vi "read_analog_inputs_from_telemetry.vi"(8 "error_in":errorcluster, 10 "channel_count":i32, 11 "paramUnicorn in":T1) -> (0 "error_out":errorcluster, 2 "values":sgl[](array[numeric]), 3 "paramUnicorn out":T1)   [LabVIEW 2017]
uses:
  Unicorn Labview Library/Control/unicorn_Param.ctl
  Unicorn Labview Library/Control/unicorn_conn.ctl
  Unicorn Labview Library/Control/unicorn_JSON.ctl
  Unicorn Labview Library/Control/unicorn_ParamInt.ctl
  Unicorn Labview Library/Control/unicorn_Telemetry.ctl
  Unicorn Labview Library/Control/unicorn_Table.ctl
  Unicorn Labview Library/Control/unicorn_ParamFloat.ctl
  Unicorn Labview Library/Unicorn Library.lvlib
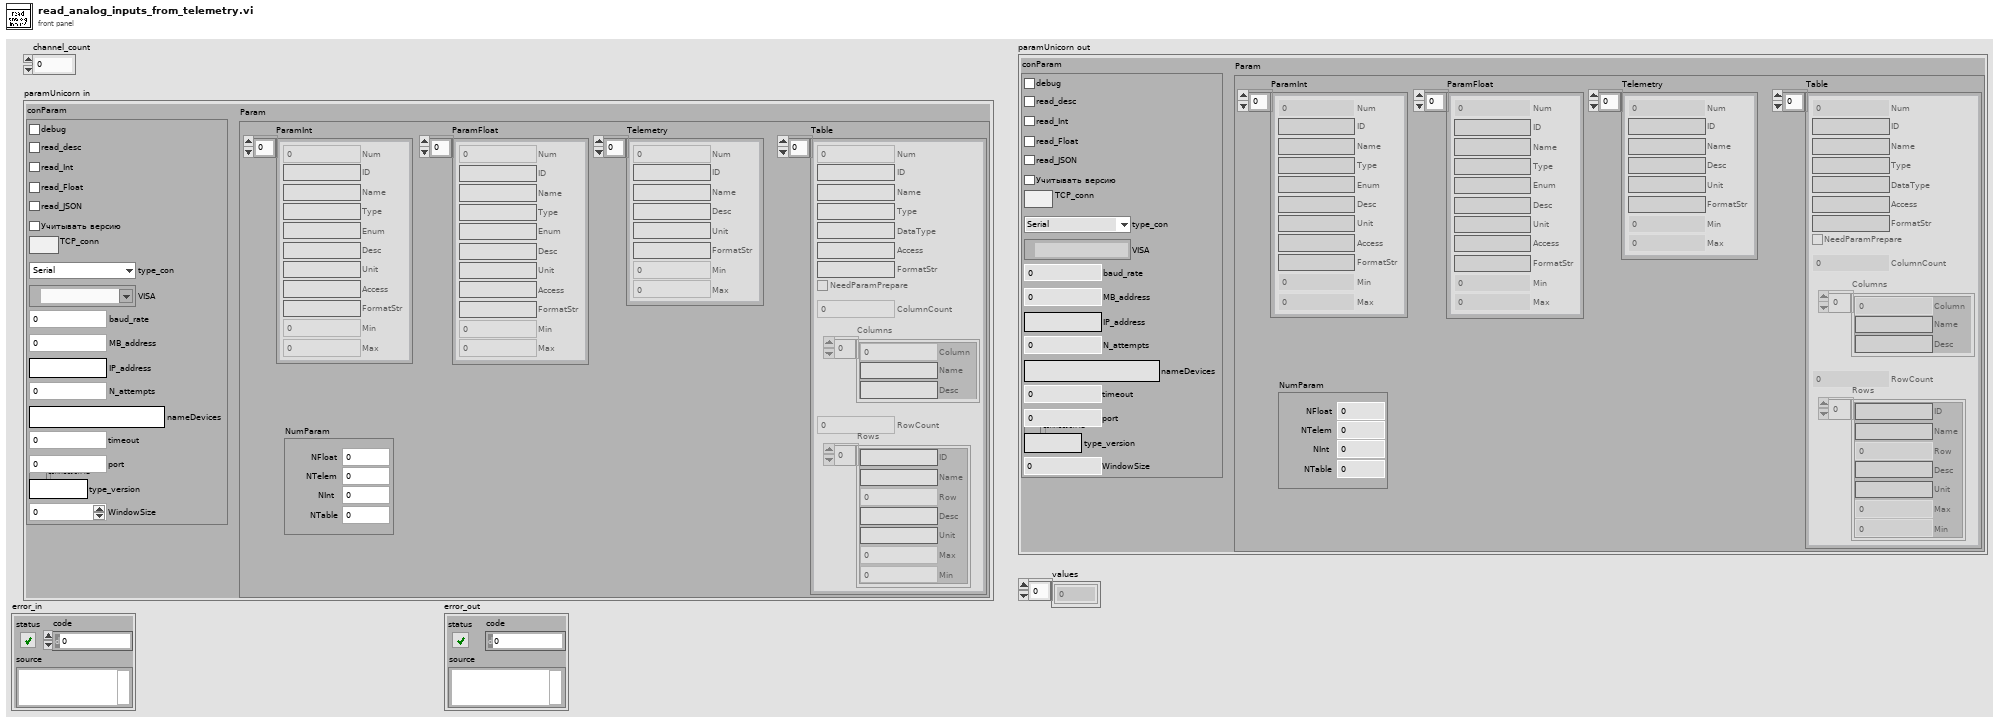
[diagram p1: front panel]
types:
  T1 = typedef "Unicorn Library.lvlib/unicorn_Param.ctl" = cluster{"conParam":T2, "Param":T3}
  T2 = typedef "Unicorn Library.lvlib/unicorn_conn.ctl" = cluster{"ReadIntParam":bool, "ReadDescrParam":bool, "ReadFloatParam":bool, "debug":bool, "ReadJSON":bool, "IP_address":string, "N_attempts":i32, "type_con":enum16{"Serial", "TCP"}, "MB_address":i32, "VISA":refnum<visa-resource-name>, "connection ID":refnum<k5>, "nameDevices":string, "timeout":i32, "port":u16, "type_version":string, "baud_rate":u32, "VersionControl":bool, "TCP_conn":bool, "WindowSize":i32}
  T3 = typedef "Unicorn Library.lvlib/unicorn_JSON.ctl" = cluster{"NumParam":cluster{"NTelem":i32, "NInt":i32, "NFloat":i32, "NTable":i32}, "ParamInt":T4, "Telemetry":T5, "Table":T6, "ParamFloat":T7}
  T4 = typedef "Unicorn Library.lvlib/unicorn_ParamInt.ctl" = cluster{"ID":string, "Num":i32, "Name":string, "Type":string, "Enum":string, "Desc":string, "Unit":string, "Access":string, "FormatStr":string, "Min":i32, "Max":i32}[]
  T5 = typedef "Unicorn Library.lvlib/unicorn_Telemetry.ctl" = cluster{"ID":string, "Num":i32, "Name":string, "Desc":string, "Unit":string, "FormatStr":string, "Min":i32, "Max":i32}[]
  T6 = typedef "Unicorn Library.lvlib/unicorn_Table.ctl" = cluster{"Num":i32, "Access":string, "ColumnCount":i32, "NeedParamPrepare":bool, "Columns":cluster{"Column":i32, "Desc":string, "Name":string}[], "DataType":string, "FormatStr":string, "ID":string, "Name":string, "RowCount":i32, "Rows":cluster{"Desc":string, "ID":string, "Max":i32, "Min":i32, "Name":string, "Row":i32, "Unit":string}[], "Type":string}[]
  T7 = typedef "Unicorn Library.lvlib/unicorn_ParamFloat.ctl" = cluster{"ID":string, "Num":i32, "Name":string, "Type":string, "Enum":string, "Desc":string, "Unit":string, "Access":string, "FormatStr":string, "Min":i32, "Max":i32}[]
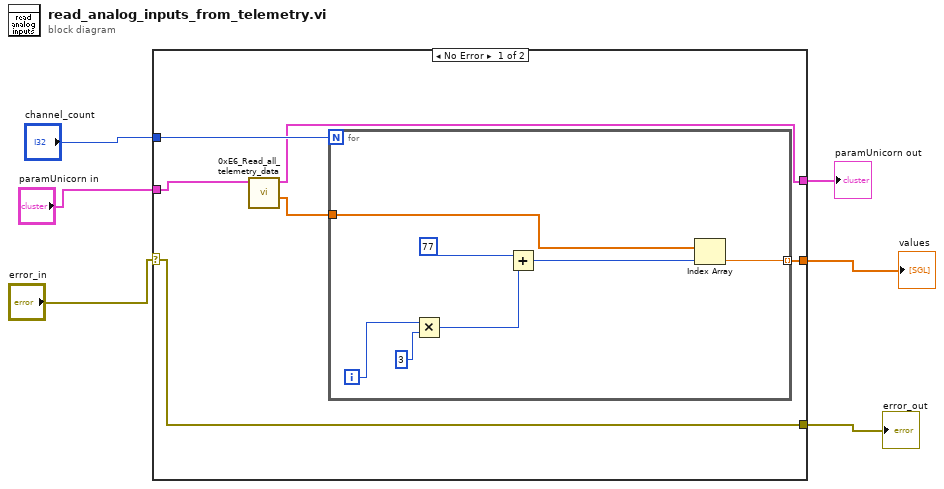
[diagram p0: block diagram]
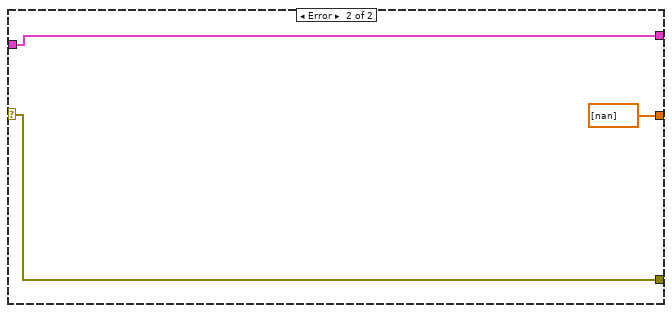
[diagram p2: hidden frame]
diagram:
  n1 = case shown="No Error" "error_in" {
    selector: "error_in" -> [w10 w21]
    tunnel: [w7 w22] -> w6
    tunnel: "paramUnicorn in" -> [w9 w22]
    tunnel: "channel_count" -> [w12 _]
    tunnel: [w11 sgl[] [nan]] -> w3
    tunnel: [w10 w21] -> w2
    frame No Error {
      n2 = call "0xE6_Read_all_telemetry_data.vi"("paramUnicorn"=w9) -> ("Telemetry"=w8:sgl[], "paramUnicorn 2"=w7:T1)  [unwired: 6 in, 2 out]
      n3 = for {
        N: w12 -> [_]
        tunnel: [w14] -> w11 mode=indexing
        tunnel: w8 -> [w13]
        i -> [w15]
        n4 = Multiply(x=w15, y=3) -> (x*y=w16:i32)
        n5 = Add(x=77, y=w16) -> (x+y=w18:i32)
        n6 = Index Array(array=w13, index=w18) -> (element=w14:sgl)
      }
    }
    frame Error {
    }
  }
  "paramUnicorn out" <- w6
  "values" <- w3
  "error_out" <- w2
